vi "Get Step Address(AC Manual).vi"(10 "Program Data.Mem Number":u32) -> (0 "Program Data.Start Address (Low)":string, 1 "Program Data.Start Address (Middle Low)":string, 2 "Program Data.Start Address (Middle High)":string, 3 "Program Data.Start Address (High)":string, 5 "Length (Low)":string, 7 "Length (High)":string)   [LabVIEW 2013]
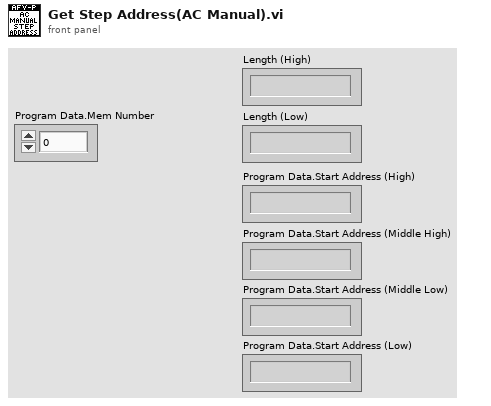
[diagram p1: front panel]
types:
  T1 = cluster{"Start Address (High)":string, "Start Address (Middle High)":string, "Start Address (Middle Low)":string, "Start Address (Low)":string, "Step Length":string, "Mem Number":u32, "Step Number":u32}
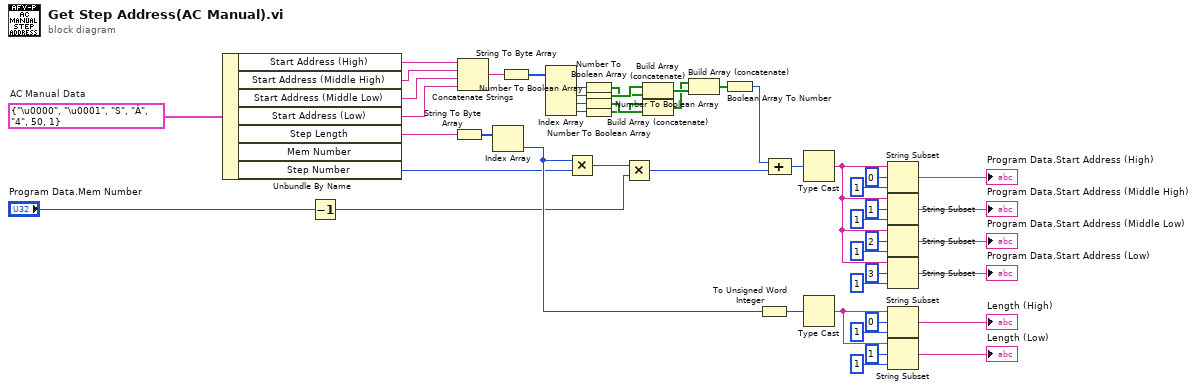
[diagram p0: block diagram]
diagram:
  w3 = T1 {"Start Address (High)"="\u0000", "Start Address (Middle High)"="\u0001", "Start Address (Middle Low)"="S", "Start Address (Low)"="Â", "Step Length"="4", "Mem Number"=50, "Step Number"=1}  # AC Manual Data
  n1 = Unbundle By Name(w3) -> ("Start Address (High)"=w8:string, "Start Address (Middle High)"=w7:string, "Start Address (Middle Low)"=w6:string, "Start Address (Low)"=w5:string, "Step Length"=w4:string, "Step Number"=w1:u32)  [unwired: 1 out]
  n2 = Decrement(x="Program Data.Mem Number") -> (x-1=w2:u32)
  n3 = String To Byte Array(string=w4) -> (unsigned byte array=w29:u8[])
  n4 = Concatenate Strings(w8, w7, w6, w5) -> (w39:string)
  n5 = Index Array(array=w29) -> (element=w9:u8)  [unwired: 1 in]
  n6 = String To Byte Array(string=w39) -> (unsigned byte array=w42:u8[])
  n7 = Index Array(array=w42) -> (element #1=w36:u8, element #2=w35:u8, element #3=w41:u8, element #4=w40:u8)  [unwired: 4 in]
  n8 = Multiply(x=w9, y=w1) -> (x*y=w11:u32)
  n9 = Number To Boolean Array(number=w36) -> (Boolean array=w33:bool[])
  n10 = Number To Boolean Array(number=w35) -> (Boolean array=w34:bool[])
  n11 = Number To Boolean Array(number=w41) -> (Boolean array=w38:bool[])
  n12 = Number To Boolean Array(number=w40) -> (Boolean array=w37:bool[])
  n13 = Multiply(x=w11, y=w2) -> (x*y=w17:u32)
  n14 = Build Array (concatenate)(w34, w33) -> (w32:bool[])
  n15 = Build Array (concatenate)(w37, w38) -> (w31:bool[])
  n16 = Build Array (concatenate)(w31, w32) -> (w30:bool[])
  n17 = Boolean Array To Number(Boolean array=w30) -> (number=w28:u32)
  n18 = To Unsigned Word Integer(number=w9) -> (unsigned 16bit integer=w10:u16)
  n19 = Compound Arithmetic op=ADD(w28, w17) -> (w18:u32)
  n20 = Type Cast(x=w18) -> (*(type *) &x=w19:string)  [unwired: 1 out]
  n21 = Type Cast(x=w10) -> (*(type *) &x=w12:string)  [unwired: 1 out]
  n22 = String Subset(string=w19, offset (0)=0, length (rest)=1 ("length (rest)")) -> (substring=→"Program Data.Start Address (High)":string)
  n23 = String Subset(string=w19, offset (0)=1, length (rest)=1 ("length (rest)")) -> (substring=→"Program Data.Start Address (Middle High)":string)
  n24 = String Subset(string=w19, offset (0)=2, length (rest)=1 ("length (rest)")) -> (substring=→"Program Data.Start Address (Middle Low)":string)
  n25 = String Subset(string=w19, offset (0)=3, length (rest)=1 ("length (rest)")) -> (substring=→"Program Data.Start Address (Low)":string)
  n26 = String Subset(string=w12, offset (0)=0, length (rest)=1 ("length (rest)")) -> (substring=→"Length (High)":string)
  n27 = String Subset(string=w12, offset (0)=1, length (rest)=1 ("length (rest)")) -> (substring=→"Length (Low)":string)
